vi "Draw.vi"(8 "error in (no error)":errorcluster, 11 "2D_Representer in":refnum<class "2D_Representer.lvclass">) -> (0 "error out":errorcluster, 2 "Display Array":u32[][](array[numeric]), 3 "2D_Representer out":refnum<class "2D_Representer.lvclass">)   [LabVIEW 2018, in "2D_Representer.lvclass"]
uses:
  2D_Representer.lvclass
  2D_Representer.lvclass/2D_Representer.ctl
  Snake/Snake.lvclass
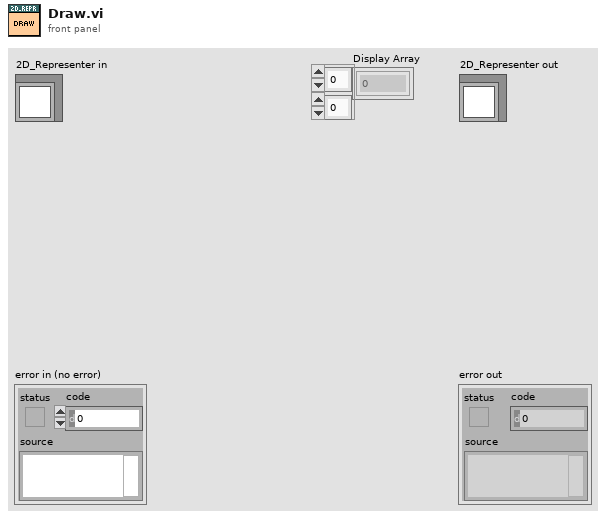
[diagram p1: front panel]
types:
  T1 = typedef "XYposition.ctl" = cluster{"Col.LocX":i32, "Row.LocY":i32}
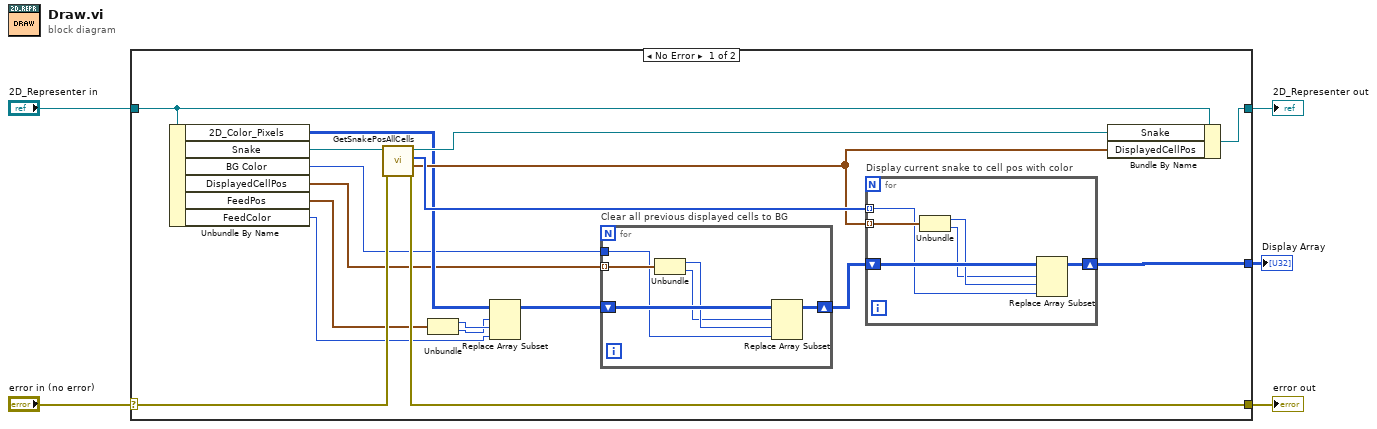
[diagram p0: block diagram]
diagram:
  n1 = case shown="No Error" "error in (no error)" {
    selector: "error in (no error)" -> [w23 w37]
    tunnel: [w22 w37] -> w4
    tunnel: [w16 w36] -> w2
    tunnel: "2D_Representer in" -> [w21 w36]
    tunnel: [w20 _] -> w1
    frame No Error {
      n2 = Unbundle By Name(w21) -> ("2D_Color_Pixels"=w14:u32[][], "Snake"=w19:refnum<class "Snake.lvclass">, "BG Color"=w12:u32, "DisplayedCellPos"=w11:T1[], "FeedPos"=w9:T1, "FeedColor"=w6:u32)
      n3 = call "GetSnakePosAllCells.vi"("error in (no error)"=w23, "Snake in"=w19) -> ("error out"=w22:errorcluster, "CellPositions"=w15:T1[], "CellColors"=w17:u32[], "Snake out"=w18:refnum<class "Snake.lvclass">)  [unwired: 6 in]
      n4 = Unbundle(w9) -> ("Col.LocX"=w8:i32, "Row.LocY"=w7:i32)
      n5 = Replace Array Subset(array=w14, new element=w6, index (row)=w7, index (col)=w8) -> (w10:u32[][])
      n6 = for "Clear all previous displayed cells to BG" {
        tunnel: w12 -> [w24]
        tunnel: w11 -> [w28] mode=indexing
        shift-right: [w27] -> w13
        shift-left: w10 -> [w29]
        n7 = Unbundle(w28) -> ("Col.LocX"=w26:i32, "Row.LocY"=w25:i32)
        n8 = Replace Array Subset(array=w29, new element=w24, index (row)=w25, index (col)=w26) -> (w27:u32[][])
      }
      n9 = for "Display current snake to cell pos with color" {
        tunnel: w17 -> [w30] mode=indexing
        tunnel: w15 -> [w34] mode=indexing
        shift-right: [w33] -> w20
        shift-left: w13 -> [w35]
        n10 = Unbundle(w34) -> ("Col.LocX"=w32:i32, "Row.LocY"=w31:i32)
        n11 = Replace Array Subset(array=w35, new element=w30, index (row)=w31, index (col)=w32) -> (w33:u32[][])
      }
      n12 = Bundle By Name(cluster=w21, "Snake"=w18, "DisplayedCellPos"=w15) -> (w16:refnum<class "2D_Representer.lvclass">)
    }
    frame Error {
    }
  }
  "error out" <- w4
  "2D_Representer out" <- w2
  "Display Array" <- w1
